vi "Friction (DBL Array).vi"(2 "offset":dbl format="%.2f", 3 "gain":dbl format="%.2f", 4 "Input Points":dbl[](array[numeric]) format="%.2f") -> (1 "Output Points":dbl[](array[numeric]) format="%.2f")   [LabVIEW 2017, in "NI_AdvCtrl_nonlinear.lvlib"]
doc: "LabVIEW no longer supports this VI. You can obtain similar functionality by installing the LabVIEW Simulation Module.\n\nRealizes a discontinuity at zero but guarantees the linear behavior elsewhere."
uses:
  <vilib>/addons/control/advanced/NI_AdvCtrl_nonlinear.lvlib
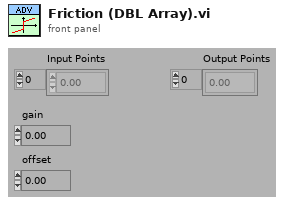
[diagram p1: front panel]
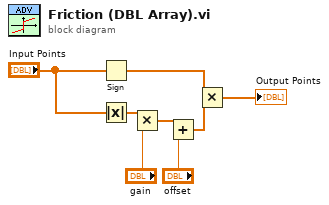
[diagram p0: block diagram]
diagram:
  n1 = Sign(1:"Input Points") -> (0:w7:dbl[])
  n2 = Absolute Value(x="Input Points") -> (abs(x)=w4:dbl[])
  n3 = Multiply(x=w4, y="gain") -> (x*y=w5:dbl[])
  n4 = Add(x=w5, y="offset") -> (x+y=w8:dbl[])
  n5 = Multiply(x=w7, y=w8) -> (x*y=→"Output Points":dbl[])
